vi "Control Type.vi"(11 "Valve in":refnum<class "HitAndHoldControl.lvclass">) -> (2 "Valve Type":string)   [LabVIEW 2020, in "VolatusControl.lvlib" / "HitAndHoldControl.lvclass"]
uses:
  HitAndHoldControl.lvclass
  HitAndHoldControl.lvclass/HitAndHoldControl.ctl
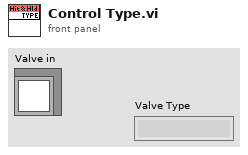
[diagram p1: front panel]
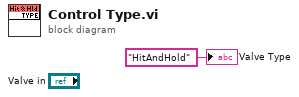
[diagram p0: block diagram]
diagram:
  "Valve Type" <- "HitAndHold" ("Valve Type")
